vi "RunTimeMenu_Save_State_TCE.vi"(8 "enabled":bool, 11 "Menu in":refnum<k9>) -> (0 "error out":errorcluster)   [LabVIEW 2020]
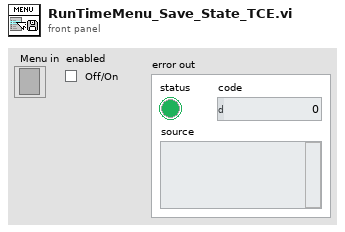
[diagram p1: front panel]
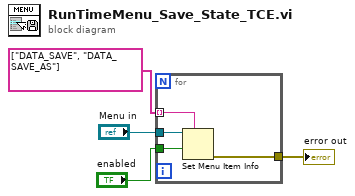
[diagram p0: block diagram]
diagram:
  n1 = for {
    tunnel: "Menu in" -> [w8]
    tunnel: string[] ["DATA_SAVE", "DATA_SAVE_AS"] ("item tag") -> [w7] mode=indexing
    tunnel: "enabled" -> [w6]
    tunnel: [w5] -> w1
    n2 = Set Menu Item Info(7:w7, 9:w6, 11:w8) -> (0:w5:errorcluster)  [unwired: 4 in, 1 out]
  }
  "error out" <- w1
